vi "Get gantry map.vi"(10 "Selection Array":dbl[](array[numeric])) -> (1 "PUT map":dbl[][](array[numeric]), 2 "Component Tray map":dbl[][](array[numeric]), 3 "Assembly Tray map":dbl[][](array[numeric]))   [LabVIEW 2018]
panel:
  out "Array":dbl[][](array[numeric])
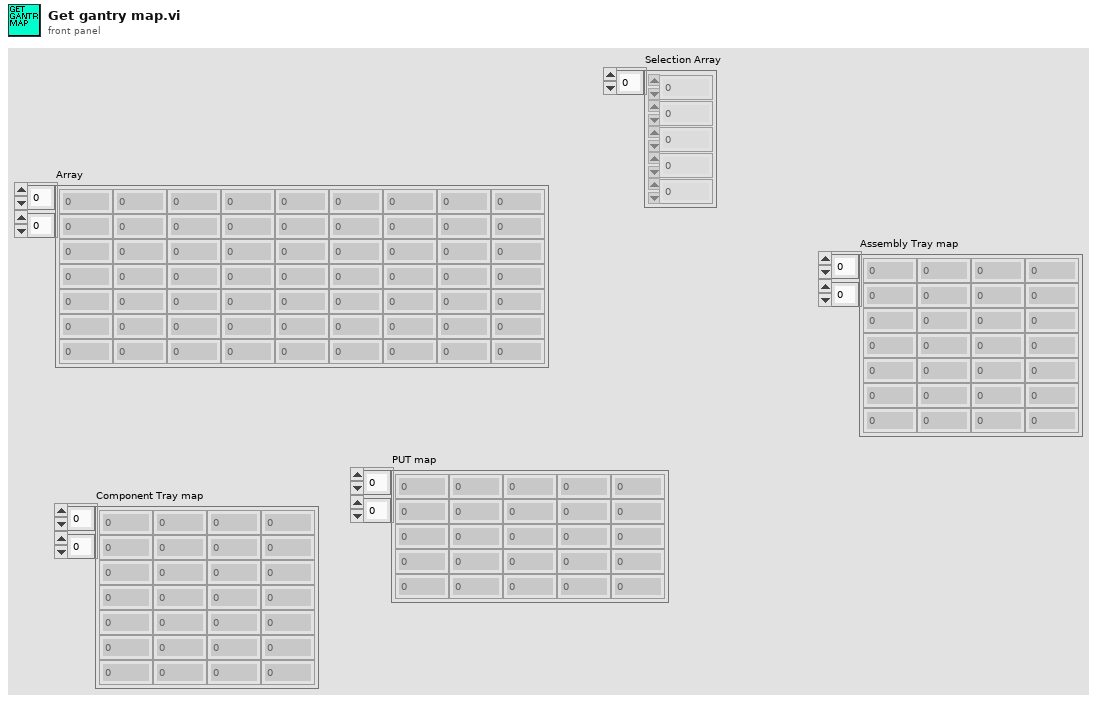
[diagram p1: front panel]
types:
  T1 = typedef "File Paths.ctl" = cluster{"Glue Pattern Folder":path, "Carrier Tray Folder":path, "Pick Up Tool Fixture Folder":path, "Components Folder":path, "Bellows Tool Offset.txt":path, "Pick Up Tool Offset.txt":path, "Dispense Tip Offset.txt":path, "Log Files":path, "Gantry Assembly Map.txt":path, "Syringe and offset map.txt":path}
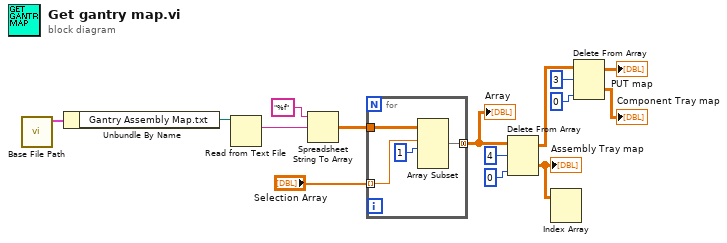
[diagram p0: block diagram]
diagram:
  n1 = call "Base File Path.vi"() -> ("Paths Out"=w2:T1)  [unwired: 11 in]
  n2 = Unbundle By Name(w2) -> ("Gantry Assembly Map.txt"=w1:path)
  n3 = Read from Text File(file (use dialog)=w1) -> (text=w15:string)  [unwired: 3 in, 3 out]
  n4 = Spreadsheet String To Array(format string="%f", spreadsheet string=w15) -> (array=w4:dbl[][])  [unwired: 2 in]
  n5 = for {
    tunnel: "Selection Array" -> [w19] mode=indexing
    tunnel: w4 -> [w18]
    tunnel: [w17] -> w3 mode=concatenating
    n6 = Array Subset(array=w18, index (row)=w19, length (row)=1) -> (w17:dbl[][])  [unwired: 2 in]
  }
  "Array" <- w3
  n7 = Delete From Array(array=w3, length=4, index (col)=0) -> (deleted portion=w8:dbl[][], array with subset deleted=w11:dbl[][])  [unwired: 1 in]
  "Assembly Tray map" <- w8
  n8 = Index Array(array=w8) -> ()  [unwired: 2 in, 1 out]
  n9 = Delete From Array(array=w11, length=3, index (col)=0) -> (deleted portion=→"Component Tray map":dbl[][], array with subset deleted=→"PUT map":dbl[][])  [unwired: 1 in]
